vi "SigInfo WfmToFreqSpectrum.vi"(8 "error in (no error)":errorcluster, 9 "SectionalSignal":waveform(sgl)) -> (0 "error out":errorcluster, 1 "MassSpectrum":cluster{"X":dbl[], "Y":sgl[]})   [LabVIEW 2018, in "SigInfo.lvclass"]
uses:
  SigInfo.lvclass
  SigInfo.lvclass/SigInfo.ctl
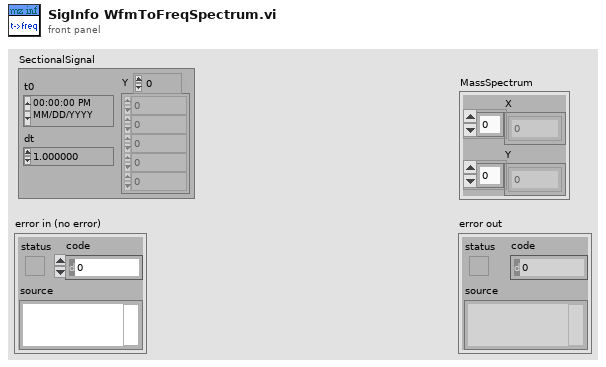
[diagram p1: front panel]
types:
  T1 = cluster{"Label":string, "dt":dbl, "Length":u32, "RefVolt":dbl, "mzTable":cluster{"t":dbl[], "mz":dbl[], "beta":dbl[]}}[]
  T2 = cluster{"Label":string, "dt":dbl, "Length":u32, "RefVolt":dbl, "mzTable":cluster{"t":dbl[], "mz":dbl[], "beta":dbl[]}}
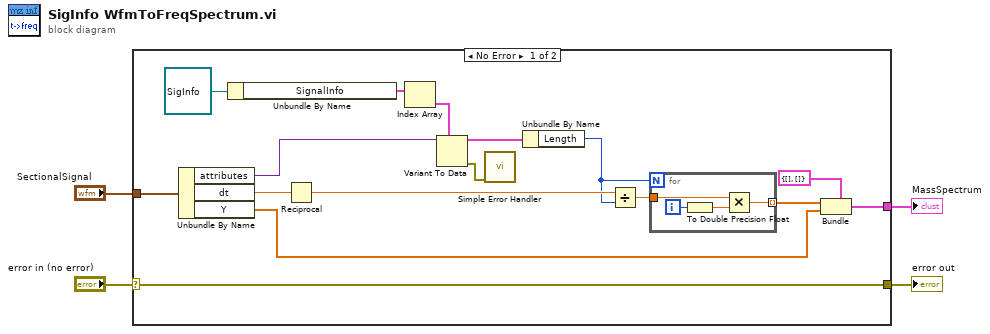
[diagram p0: block diagram]
diagram:
  n1 = case shown="No Error" "error in (no error)" {
    selector: "error in (no error)" -> [w20 w25]
    tunnel: [w20 w25] -> w3
    tunnel: "SectionalSignal" -> [w19 _]
    tunnel: [w5 _] -> w1
    frame No Error {
      n2 = Unbundle By Name(w19) -> ("attributes"=w14:variant, "dt"=w18:dbl, "Y"=w6:sgl[])
      n3 = Unbundle By Name(refnum<class "SigInfo.lvclass"> refnum ("SigInfo.lvclass")) -> ("SignalInfo"=w16:T1)
      n4 = Reciprocal(x=w18) -> (1/x=w11:dbl)
      n5 = Index Array(array=w16) -> (element=w15:T2)  [unwired: 1 in]
      n6 = Variant To Data(type=w15, Variant=w14) -> (data=w12:T2, error out=w13:errorcluster)  [unwired: 1 in]
      n7 = call <vilib>:"Simple Error Handler.vi"("error in (no error)"=w13) -> ()  [unwired: 4 in, 5 out]
      n8 = Unbundle By Name(w12) -> ("Length"=w10:u32)
      n9 = Divide(x=w11, y=w10) -> (x/y=w9:dbl)
      n10 = for {
        N: w10 -> [_]
        tunnel: w9 -> [w22]
        tunnel: [w21] -> w7 mode=indexing
        i -> [w24]
        n11 = To Double Precision Float(number=w24) -> (double precision float=w23:dbl)
        n12 = Multiply(x=w22, y=w23) -> (x*y=w21:dbl)
      }
      n13 = Bundle(cluster=cluster{"X":dbl[], "Y":sgl[]} {"X"=[], "Y"=[]} ("MassSpectrum 2"), "X"=w7, "Y"=w6) -> (w5:cluster{"X":dbl[], "Y":sgl[]})
    }
    frame Error {
    }
  }
  "error out" <- w3
  "MassSpectrum" <- w1
